vi "Camera Update Slider Limits.vi"(0 "Refnums":refnum<vi>[](array[refnum]), 1 "Edit?":T1(ring), 5 "Data Entry Limits:Increment":dbl, 7 "Data Entry Limits:Maximum":dbl, 9 "Data Entry Limits:Minimum":dbl, 11 "error in (no error)":errorcluster, 12 "Disabled":u8, 13 "Value":variant) -> (15 "error out":errorcluster)   [LabVIEW 2014]
panel:
  # "LICENSED MATERIALS – PROPERTY OF IBM\nCopyright IBM Corp. 2016,\nALL RIGHTS RESERVED"
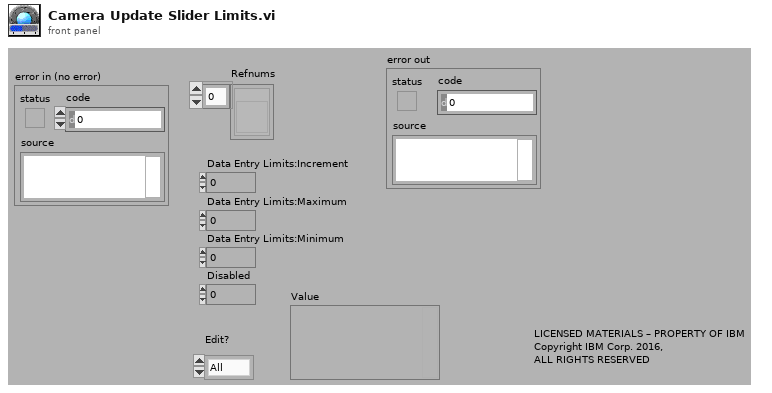
[diagram p1: front panel]
types:
  T1 = enum16{"All", "Limits", "Value", "User Enablement"}
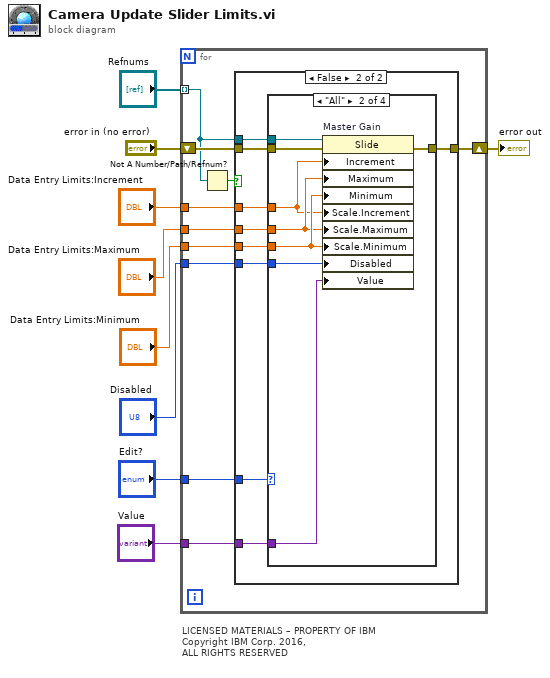
[diagram p0: block diagram]
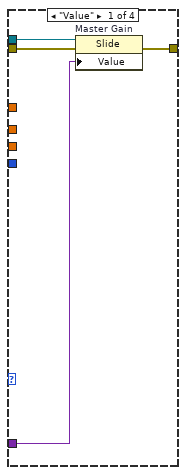
[diagram p3: hidden frame]
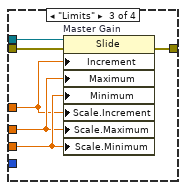
[diagram p4: hidden frame]
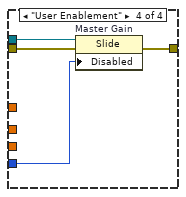
[diagram p5: hidden frame]
diagram:
  # "LICENSED MATERIALS – PROPERTY OF IBM\nCopyright IBM Corp. 2016,\nALL RIGHTS RESERVED"
  n1 = for {
    tunnel: "Refnums" -> [w12] mode=indexing
    shift-right: [w18] -> w8
    shift-left: "error in (no error)" -> [w19]
    tunnel: "Disabled" -> [w17]
    tunnel: "Data Entry Limits:Minimum" -> [w16]
    tunnel: "Data Entry Limits:Maximum" -> [w15]
    tunnel: "Data Entry Limits:Increment" -> [w14]
    tunnel: "Edit?" -> [w11]
    tunnel: "Value" -> [w10]
    n2 = Not A Number/Path/Refnum?(number/path/refnum=w12) -> (NaN/Path/Refnum?=w13:bool)
    n3 = case shown="False" w13 {
      tunnel: w19 -> [w20 w29]
      tunnel: [w20 w28] -> w18
      tunnel: w12 -> [_ w27]
      tunnel: w17 -> [_ w26]
      tunnel: w16 -> [_ w25]
      tunnel: w15 -> [_ w24]
      tunnel: w14 -> [_ w23]
      tunnel: w11 -> [_ w22]
      tunnel: w10 -> [_ w21]
      frame True {
      }
      frame False {
        n4 = case shown="\"All\"" w22 {
          tunnel: w29 -> [w33 w41 w47 w51]
          tunnel: [w32 w40 w46 w50] -> w28
          tunnel: w27 -> [w31 w39 w45 w49]
          tunnel: w26 -> [_ w38 _ w48]
          tunnel: w25 -> [_ w37 w44 _]
          tunnel: w24 -> [_ w36 w43 _]
          tunnel: w23 -> [_ w35 w42 _]
          tunnel: w21 -> [w30 w34 _ _]
          frame "Value" {
            n5 = property on="Master Gain" class="Slide"(reference=w31, error in=w33, "Value"=w30) -> (error out=w32:errorcluster)  [unwired: 1 out]
          }
          frame "All" {
            n6 = property on="Master Gain" class="Slide"(reference=w39, error in=w41, "Increment"=w35, "Maximum"=w36, "Minimum"=w37, "Scale.Increment"=w35, "Scale.Maximum"=w36, "Scale.Minimum"=w37, "Disabled"=w38, "Value"=w34) -> (error out=w40:errorcluster)  [unwired: 1 out]
          }
          frame "Limits" {
            n7 = property on="Master Gain" class="Slide"(reference=w45, error in=w47, "Increment"=w42, "Maximum"=w43, "Minimum"=w44, "Scale.Increment"=w42, "Scale.Maximum"=w43, "Scale.Minimum"=w44) -> (error out=w46:errorcluster)  [unwired: 1 out]
          }
          frame "User Enablement" {
            n8 = property on="Master Gain" class="Slide"(reference=w49, error in=w51, "Disabled"=w48) -> (error out=w50:errorcluster)  [unwired: 1 out]
          }
        }
      }
    }
  }
  "error out" <- w8
